vi "Setup.vi"(8 "error in (no error)":errorcluster, 11 "Compiled Data In":T1={"Name"="", "Async Init Timeout"=0, "Segment Files"=FALSE, "Segment Every"=0.0, "Segment by"=enum."Size (MB)", "dt per loop"=0.0, "output cluster"={"Name"="", "Directory"="", "Date Captured"="", "Groups"=[], "Meta Data"=[], "File Start Time"=timestamp(0 s since 1904-01-01), "appended path"=path ""}} {"output cluster"."Groups"."Channels"."Data Reference" format="%.0x"}) -> (0 "error out":errorcluster, 3 "Channel Manager out":refnum<class "Channel Manager.lvclass">)   [LabVIEW 2024, in "Embedded TDMS Logger Engine.lvlib" / "Channel Manager.lvclass"]
doc: "Start by creating our File Class and instantiating it from our Compiled Settings data."
uses:
  Channel Manager.lvclass
  Shared/Compiled.Settings.ctl
  Shared/SegmentOptions.ctl
  Shared/File Classes/File/FileAsCluster.ctl
  Shared/File Classes/Group/GroupAsCluster.ctl
  Shared/File Classes/Channel/ChannelAsCluster.ctl
  <vilib>/NI VeriStand/Custom Device API/Data Reference.ctl
  Shared/File Classes/Meta Data.ctl
  Channel Manager.lvclass/Channel Manager.ctl
  Shared/File Classes/File/File.lvclass
  Shared/Embedded TDMS Logger Shared.lvlib
  <vilib>/NI VeriStand/Custom Device API/Custom Device API.lvlib
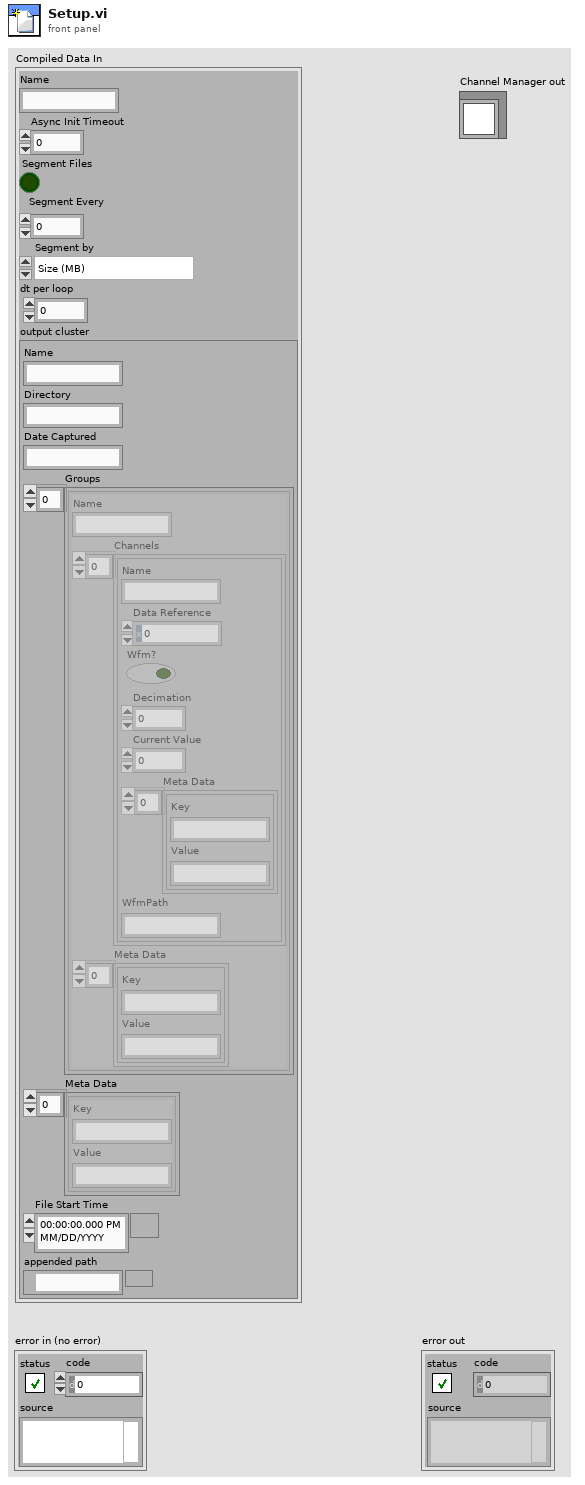
[diagram p1: front panel]
types:
  T1 = typedef "Embedded TDMS Logger Shared.lvlib/Compiled.Settings.ctl" = cluster{"Name":string, "Async Init Timeout":u16, "Segment Files":bool, "Segment Every":dbl, "Segment by":T2, "dt per loop":dbl, "output cluster":T3}
  T2 = typedef "SegmentOptions.ctl" = enum16{"Time (s)", "Size (MB)"}
  T3 = typedef "FileAsCluster.ctl" = cluster{"Name":string, "Directory":string, "Date Captured":string, "Groups":T4[], "Meta Data":T7[], "File Start Time":timestamp, "appended path":path}
  T4 = typedef "GroupAsCluster.ctl" = cluster{"Name":string, "Channels":T5[], "Meta Data":T7[]}
  T5 = typedef "ChannelAsCluster.ctl" = cluster{"Name":string, "Data Reference":T6, "Wfm?":bool, "Decimation":i32, "Current Value":dbl, "Meta Data":T7[], "WfmPath":string}
  T6 = typedef "Custom Device API.lvlib/Data Reference.ctl" = i32
  T7 = typedef "Meta Data.ctl" = cluster{"Key":string, "Value":string}
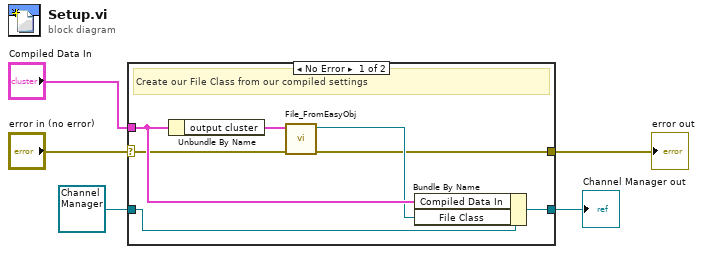
[diagram p0: block diagram]
diagram:
  n1 = case shown="No Error" "error in (no error)" {
    selector: "error in (no error)" -> [w8 w14]
    tunnel: [w6 w14] -> w4
    tunnel: [w11 w13] -> w3
    tunnel: refnum<class "Channel Manager.lvclass"> refnum ("Channel Manager in") -> [w12 w13]
    tunnel: "Compiled Data In" -> [w9 _]
    frame No Error {
      # "Create our File Class from our compiled settings"
      n2 = Unbundle By Name(w9) -> ("output cluster"=w10:T3)
      n3 = call "File_FromEasyObj.vi"("error in (no error)"=w8, "output cluster"=w10) -> ("error out"=w6:errorcluster, "File out"=w7:refnum<class "File.lvclass">)  [unwired: 8 in]
      n4 = Bundle By Name(cluster=w12, "Compiled Data In"=w9, "File Class"=w7) -> (w11:refnum<class "Channel Manager.lvclass">)
    }
    frame Error {
    }
  }
  "error out" <- w4
  "Channel Manager out" <- w3
